vi "Obtain Default Broadcast Events.vi"(8 "error in":errorcluster) -> (0 "error out":errorcluster, 1 "Update Module Execution Status":refnum<user-event>, 2 "Error Reported":refnum<user-event>, 3 "Status Updated":refnum<user-event>, 4 "System Message":refnum<user-event>, 5 "Module Did Stop":refnum<user-event>)   [LabVIEW 2020, in "DBModule.lvlib"]
doc: "____\nHAMPEL SOFTWARE ENGINEERING v2.6.0 (2023-12-19 10:54)"
uses:
  DBModule.lvlib
  Status Updated Argument--cluster.ctl
  Error Reported Argument--cluster.ctl
  Stop Argument--cluster.ctl
  Get Module Execution Status Argument--cluster.ctl
  System Message Argument--cluster.ctl
  Libraries/hse-libraries/Source/hse-dqmh/Controls/System Message Source.ctl
  Libraries/hse-libraries/Source/hse-dqmh/hse-dqmh.lvlib
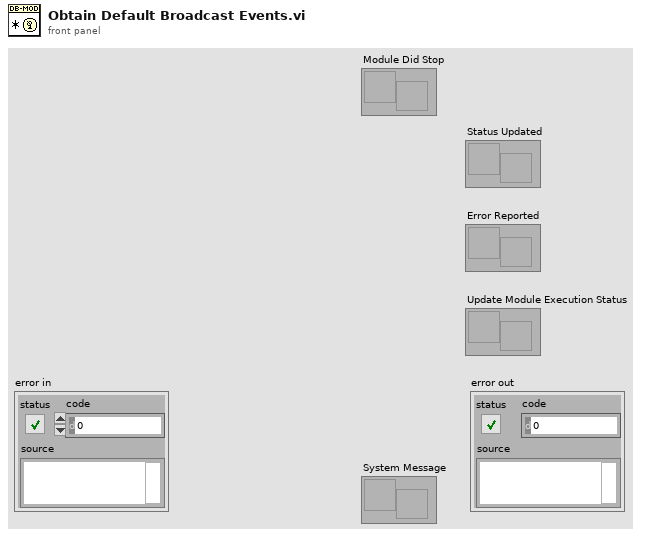
[diagram p1: front panel]
types:
  T1 = typedef "DBModule.lvlib/Broadcast Events--cluster.ctl" = cluster{"Module Did Init":refnum<user-event>, "Status Updated":refnum<user-event>, "Error Reported":refnum<user-event>, "Module Did Stop":refnum<user-event>, "Update Module Execution Status":refnum<user-event>, "System Message":refnum<user-event>}
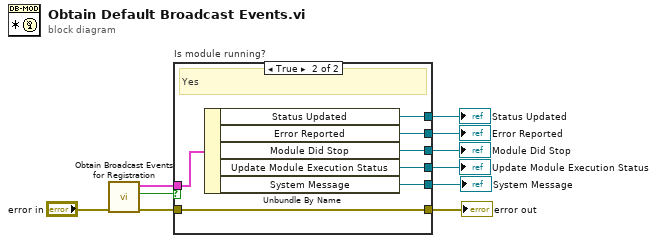
[diagram p0: block diagram]
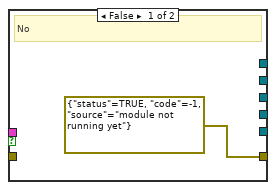
[diagram p2: hidden frame]
diagram:
  n1 = call "Obtain Broadcast Events for Registration.vi"("error in (no error)"="error in") -> ("error out"=w2:errorcluster, "Already running?"=w3:bool, "DBModule Broadcast Events"=w9:T1)  [unwired: 8 in]
  n2 = case "Is module running?" shown="True" w3 {
    tunnel: w9 -> [_ w18]
    tunnel: [_ w17] -> w8
    tunnel: [_ w16] -> w7
    tunnel: [_ w15] -> w6
    tunnel: [_ w14] -> w5
    tunnel: [_ w13] -> w4
    tunnel: w2 -> [_ w12]
    tunnel: [errorcluster {"status"=TRUE, "code"=-1, "source"="module not running yet"} ("error out") w12] -> w1
    frame False {
      # "No"
    }
    frame True {
      # "Yes"
      n3 = Unbundle By Name(w18) -> ("Status Updated"=w17:refnum<user-event>, "Error Reported"=w16:refnum<user-event>, "Module Did Stop"=w15:refnum<user-event>, "Update Module Execution Status"=w14:refnum<user-event>, "System Message"=w13:refnum<user-event>)
    }
  }
  "error out" <- w1
  "Status Updated" <- w8
  "Error Reported" <- w7
  "Module Did Stop" <- w6
  "Update Module Execution Status" <- w5
  "System Message" <- w4
